vi "Furnace 2016.vi"() -> ()   [LabVIEW 2015]
panel:
  in  "Numeric 2":dbl
  in  "Numeric":dbl
  out "Off":bool
  in  "Thermometer":dbl(slide) scale=0.0..100.0
  out "On":bool
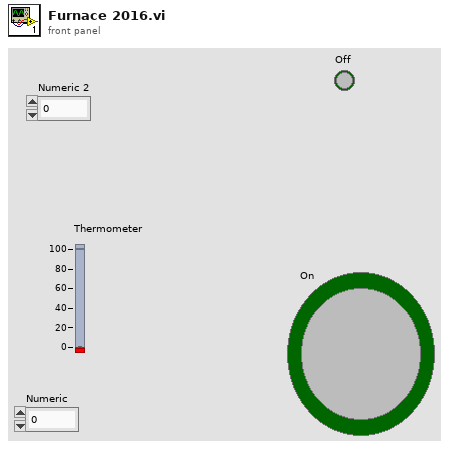
[diagram p1: front panel]
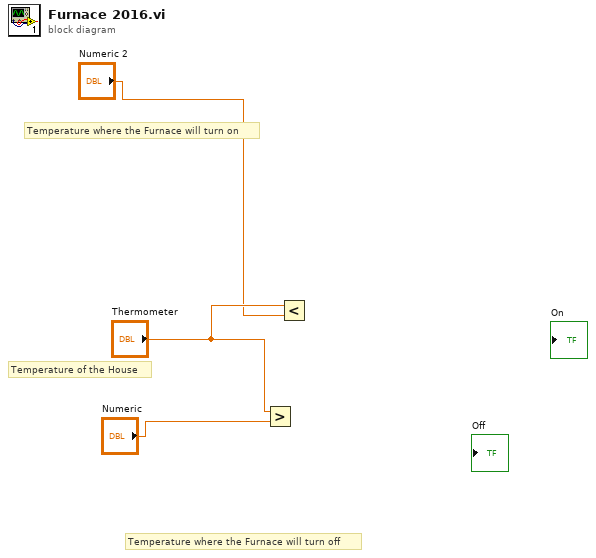
[diagram p0: block diagram]
diagram:
  # "Temperature of the House"
  # "Temperature where the Furnace will turn off"
  # "Temperature where the Furnace will turn on"
  n1 = Greater?(x="Thermometer", y="Numeric") -> ()  [unwired: 1 out]
  n2 = Less?(x="Thermometer", y="Numeric 2") -> ()  [unwired: 1 out]
